vi "Msg_BuildSystemMsg.vi"(0 "ListBoxRef":refnum<vi>, 1 "LogType":T2=enum."Manual", 5 "Data":string, 7 "Time":string, 9 "MsgPageSelect":T1=enum."Action", 11 "User":string) -> ()   [LabVIEW 2019, in "MsgShowAndLog.lvlib"]
uses:
  MsgShowAndLog.lvlib
  Ctrl/MsgTyp.ctl
  Ctrl/LogType.ctl
  Ctrl/MsgPageSelect.ctl
panel:
  in  "Type":T3
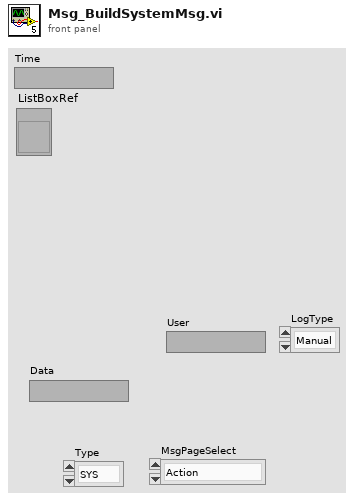
[diagram p1: front panel]
types:
  T1 = typedef "MsgShowAndLog.lvlib/MsgPageSelect.ctl" = enum16{"System", "Comm", "IO", "Action", "Alarm"}
  T2 = typedef "MsgShowAndLog.lvlib/LogType.ctl" = enum16{"Auto", "Manual", "Handshake", "Error"}
  T3 = typedef "MsgShowAndLog.lvlib/MsgTyp.ctl" = enum16{"SYS", "COMM", "IO", "Action", "Alarm"}
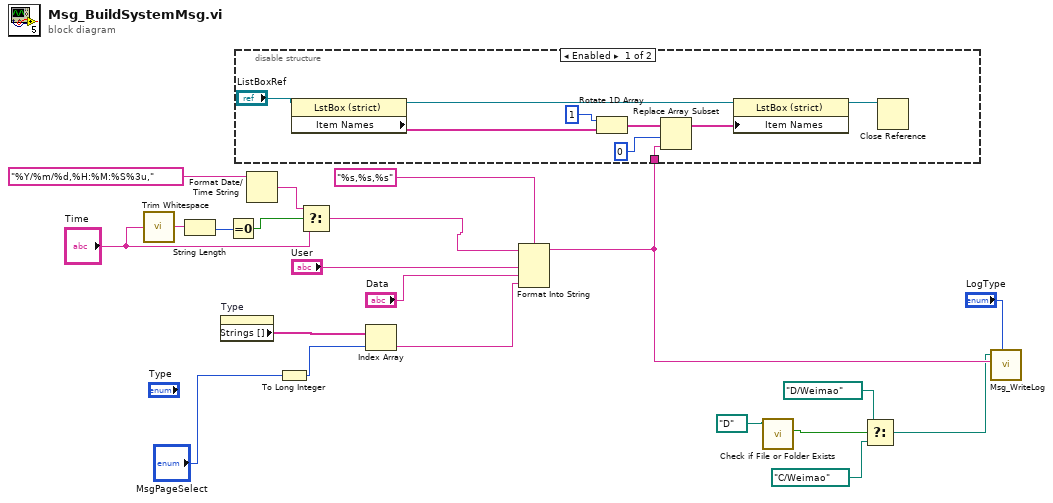
[diagram p0: block diagram]
diagram:
  n1 = call <vilib>:"Trim Whitespace.vi"("string"="Time") -> ("trimmed string"=w9:string)  [unwired: 1 in]
  n2 = String Length(string=w9) -> (length=w8:i32)
  n3 = property on="Type" class="Enum (strict)"() -> ("Strings []"=w20:string[])  [unwired: 2 in, 2 out]
  n4 = Equal To 0?(x=w8) -> (x = 0?=w7:bool)
  n5 = Format Date/Time String(time format string (%c)="%Y/%m/%d,%H:%M:%S%3u,") -> (date/time string=w12:string)  [unwired: 2 in]
  n6 = To Long Integer(number="MsgPageSelect") -> (32bit integer=w19:i32)
  n7 = Select(t=w12, s=w7, f="Time") -> (s? t:f=w11:string)
  n8 = Index Array(array=w20, index=w19) -> (element=w16:string)
  n9 = Format Into String(format string="%s,%s,%s", initial string=w11, "User", "Data", w16) -> (resulting string=w15:string)  [unwired: 1 in, 1 out]
  n10 = disable-structure shown="Enabled" {
    disable-tunnel: w15 -> [w23 _]
    frame Enabled {
      n11 = property class="LstBox (strict)"(reference="ListBoxRef") -> (reference out=w25:refnum<vi>, "Item Names"=w27:string[])  [unwired: 1 in, 1 out]
      n12 = Rotate 1D Array(1:w27, 2:1 ("n")) -> (0:w29:string[])
      n13 = Replace Array Subset(array=w29, new element=w23, index=0) -> (w26:string[])
      n14 = property class="LstBox (strict)"(reference=w25, "Item Names"=w26) -> (reference out=w24:refnum<vi>)  [unwired: 1 in, 1 out]
      n15 = Close Reference(reference=w24) -> ()  [unwired: 1 in, 1 out]
    }
    frame Disabled {
    }
  }
  n16 = call <vilib>:"Check if File or Folder Exists.vi"("path"=path "D:/" ("Base Path")) -> ("file or folder exists?"=w5:bool)  [unwired: 8 in, 2 out]
  n17 = Select(t=path "D:/Weimao" ("Base Path"), s=w5, f=path "C:/Weimao" ("Base Path")) -> (s? t:f=w3:path)
  n18 = call "Msg_WriteLog.vi"("LogType"="LogType", "Text"=w15, "Base Path"=w3) -> ()  [unwired: 8 in, 1 out]
